vi "TAI_Solenoid.vi"(2 "Normal Output":bool, 3 "Actuator Name":string) -> (0 "Interlock Output":bool, 1 "Testing This Actuator":bool)   [LabVIEW 2019]
doc: "This VI functions as an interlock, allowing operators to bypass the control logic for each actuator and test it using basic commands. This VI supports both floating point and boolean outputs. It requires integration with global variables storing the test signal and the operator's actuator selection. It is intended to integrate with the standard FRC 4265 control architecture."
uses:
  dsdata.vi
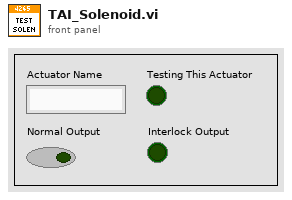
[diagram p1: front panel]
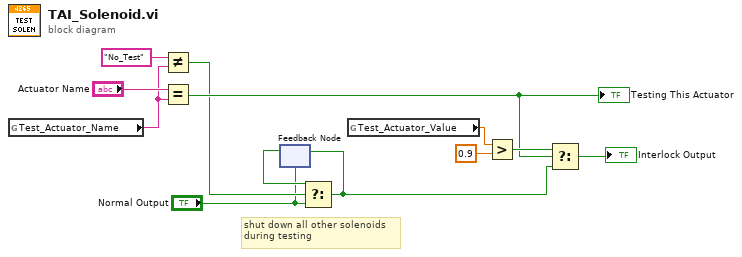
[diagram p0: block diagram]
diagram:
  # "shut down all other solenoids\nduring testing"
  n1 = global read "dsdata.vi" "Test_Actuator_Name"() -> (w2:string)
  n2 = Not Equal?(x="No_Test", y=w2) -> (x != y?=w3:bool)
  n3 = Equal?(x="Actuator Name", y=w2) -> (x = y?=w8:bool)
  "Testing This Actuator" <- w8
  n4 = feedback #1("Normal Output") -> (w4:bool)
  n5 = Select(t=w4, s=w3, f="Normal Output") -> (s? t:f=w5:bool)
  n6 = feedback-in #1(w5) -> ()
  n7 = global read "dsdata.vi" "Test_Actuator_Value"() -> (w12:dbl)
  n8 = Greater?(x=w12, y=0.9) -> (0:w10:bool)
  n9 = Select(t=w10, s=w8, f=w5) -> (s? t:f=→"Interlock Output":bool)
